vi "CONFIG-SET.vi"(0 "TCP session out":refnum<k5>, 5 "Parameter":string, 7 "Value":string, 11 "error in":errorcluster) -> (4 "TCP session out":refnum<k5>, 6 "Data":T1, 15 "error out":errorcluster)   [LabVIEW 2023]
uses:
  SubVIs/Controls/redis-data.ctl
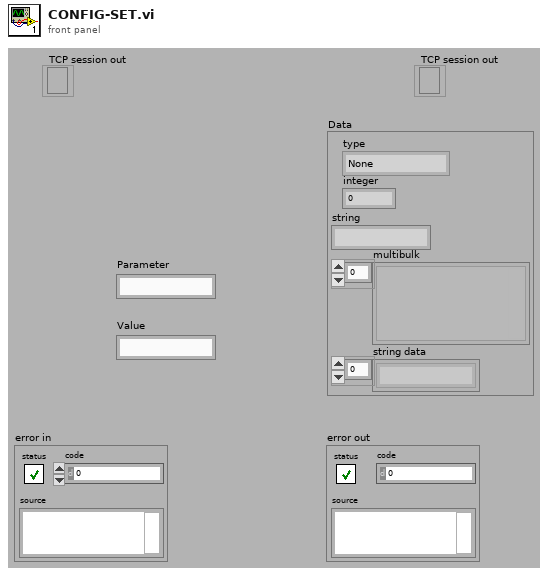
[diagram p1: front panel]
types:
  T1 = typedef "redis-data.ctl" = cluster{"type":enum16{"None", "Error", "Status", "Nil", "Integer", "String", "Multibulk"}, "integer":i64, "string":string, "multibulk":variant[], "string data":string[]}
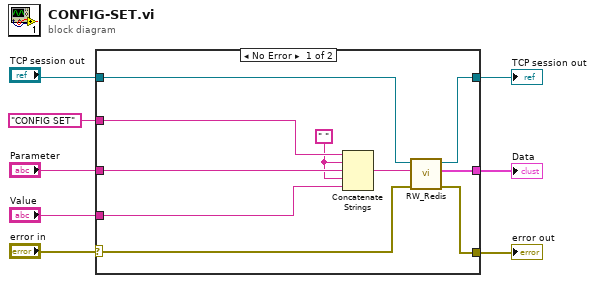
[diagram p0: block diagram]
diagram:
  n1 = case shown="No Error" "error in" {
    selector: "error in" -> [w16 w20]
    tunnel: "Parameter" -> [w13 _]
    tunnel: "CONFIG SET" -> [w18 _]
    tunnel: "TCP session out" -> [w10 w19]
    tunnel: [w15 w20] -> w6
    tunnel: [w14 _] -> w1
    tunnel: "Value" -> [w11 _]
    tunnel: [w9 w19] -> w2
    frame No Error {
      w12 = " "
      n2 = Concatenate Strings(w18, w12, w13, w12, w11) -> (w17:string)
      n3 = call "RW_Redis.vi"("error in"=w16, "command"=w17, "TCP session in"=w10) -> ("error out"=w15:errorcluster, "Data"=w14:T1, "TCP session out"=w9:refnum<k5>)  [unwired: 6 in]
    }
    frame Error {
    }
  }
  "error out" <- w6
  "Data" <- w1
  "TCP session out" <- w2
